vi "dspMult_32x32.vi"(6 "sclr":bool, 8 "b":fxp<+/-,32,5>, 11 "a":fxp<+/-,32,5>) -> (2 "p":fxp<+/-,64,10>)   [LabVIEW 2017]
doc: "32x32 multiplier.\nUses 1 dsp block\nHas 8 cycles of latency.\n5 integer bits on both inputs, 10 integer bits on output"
uses:
  <vilib>/rvi/IPIntegrationNode/IPINode_Typedef/niFpgaIPINodeSupportedFamilies.ctl
  <vilib>/rvi/IPIntegrationNode/IPINode_Utilities/niFpgaIPINodeSimCore.vi
  <vilib>/rvi/XilinxIP/XIPIN_XNode/niFpgaXIPIN.xnode
  dspMult_32x32/Multiplier 1/Multiplier_1_87D7BDF9F83143F1B5E978F9A992495A.dll
  <vilib>/rvi/IPIntegrationNode/IPINode_Xnode/niFpgaIPINode.xnode
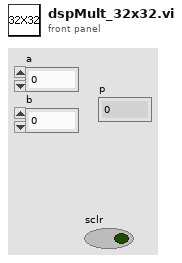
[diagram p1: front panel]
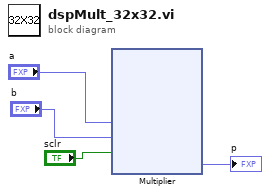
[diagram p0: block diagram]
diagram:
  n1 = xnode ("Multiplier")("a"="a", "b"="b", "sclr"="sclr") -> ("p"=→"p":fxp<+/-,64,10>)  [unwired: 1 in]
